vi "UIDetectClickedSquare.vi"(11 "Array in":refnum<vi>) -> (0 "error out":errorcluster, 3 "Map":map{string, i32}(c390))   [LabVIEW 2020]
uses:
  <vilib>/Utility/miscctls.llb/LVBoundsTypeDef.ctl
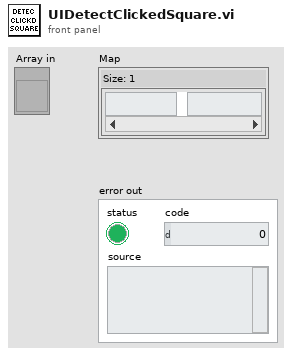
[diagram p1: front panel]
types:
  T1 = typedef "LVBoundsTypeDef.ctl" = cluster{"Width":u32, "Height":u32}
  T2 = typedef "LVPositionTypeDef.ctl" = cluster{"Left":i32, "Top":i32}
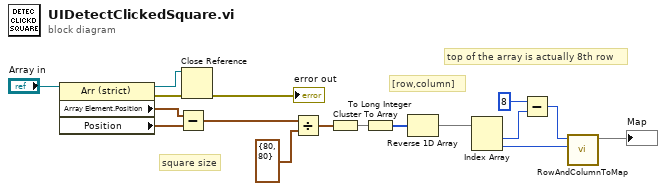
[diagram p0: block diagram]
diagram:
  # "top of the array is actually 8th row"
  # "[row,column]"
  # "square size"
  n1 = property class="Arr (strict)"(reference="Array in") -> (reference out=w7:refnum<vi>, error out=w10:errorcluster, "Array Element.Position"=w11:T2, "Position"=w13:T2)  [unwired: 1 in]
  n2 = Subtract(x=w11, y=w13) -> (x-y=w12:T2)
  n3 = Close Reference(reference=w7, error in (no error)=w10) -> (error out=→"error out":errorcluster)
  n4 = Divide(x=w12, y=T1 {"Width"=80, "Height"=80}) -> (x/y=w15:cluster{dbl, dbl})
  n5 = Cluster To Array(cluster=w15) -> (array=w16:dbl[])
  n6 = To Long Integer(number=w16) -> (32bit integer=w17:i32[])
  n7 = Reverse 1D Array(array=w17) -> (reversed array=w4:i32[])
  n8 = Index Array(array=w4) -> (element #1=w3:i32, element #2=w5:i32)  [unwired: 2 in]
  n9 = Subtract(x=8, y=w3) -> (x-y=w1:i32)
  n10 = call "RowAndColumnToMap.vi"("Column"=w5, "Row"=w1) -> ("map"=→"Map":map{string, i32})  [unwired: 9 in]
